vi "Get parameters from filename.vi"(0 "Filename":string="WS1021_PCB_01-03_VDD2p50CP17_R2-074200_R3-074302.s2p_right_DUT", 1 "File name format":T1, 3 "Comment lines":string[](array[string]), 5 "Idd":dbl, 9 "extension":string, 11 "Error In":errorcluster) -> (4 "Heading":string[](array[string]), 6 "Info":string[](array[string]), 10 "Registers":string[][](array[string]), 12 "Vdd (V)":dbl, 15 "Error Out":errorcluster)   [LabVIEW 2020]
uses:
  File Name Format.ctl
panel:
  out "CPV 2":i32(ring)=17 items=["CP 24V", "CP 26V", "CP 28V", "CP 30V", "CP 31V", "CP 32V", "CP 33V", "CP 34V", "CP 35V", "CP 36V", "CP 37V", "CP 38V", "CP 39V", "CP 40V", "CP 41V", "CP 42V", "CP 43V", "CP 44V", "CP 45V", "CP 46V", "CP 47V", "CP 48V", "CP 49V", "CP 50V", "CP 51V", "CP 52V", "CP 53V", "CP 54V", "CP 56V", "CP 58V", "CP 60V", "CP 62V"]
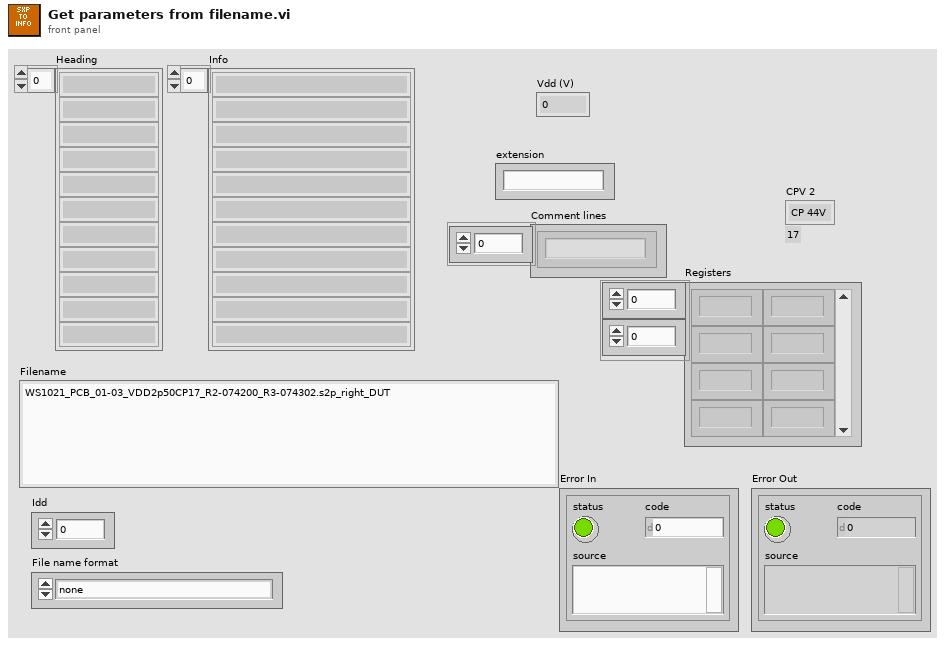
[diagram p1: front panel]
types:
  T1 = typedef "File Name Format.ctl" = enum16{"none", "S-para, old", "S-para, new", "S-para, new, step", "ECP", "S-para, new+1", "WS1040", "S-para, new+5100", "S-para, new+5100, no step", "General, space limited", "General, underscore limited", "General, whitespace limited", "LV-framework", "LV-framework, no file name"}
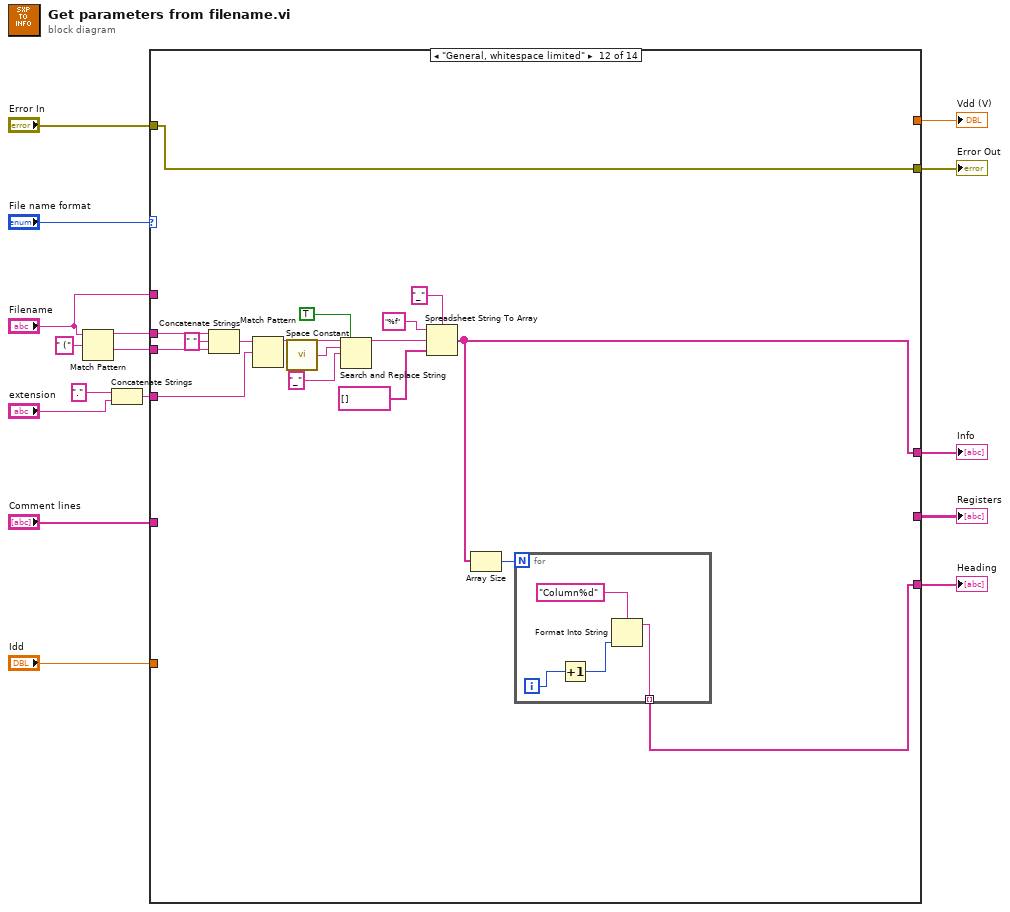
[diagram p0: block diagram]
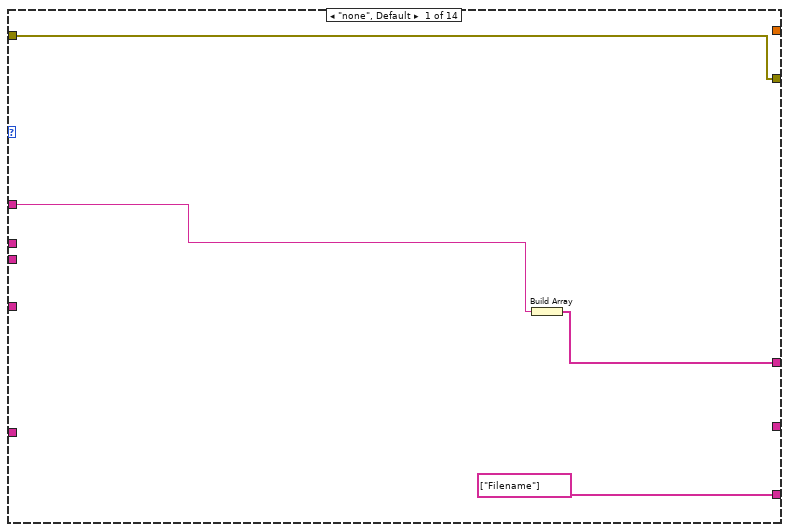
[diagram p2: hidden frame]
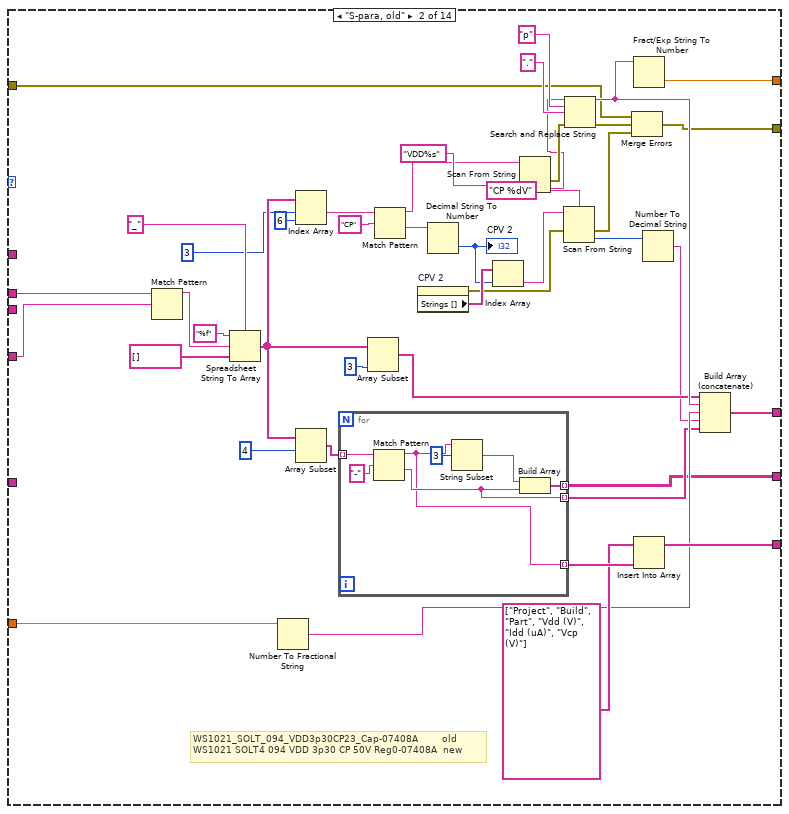
[diagram p3: hidden frame]
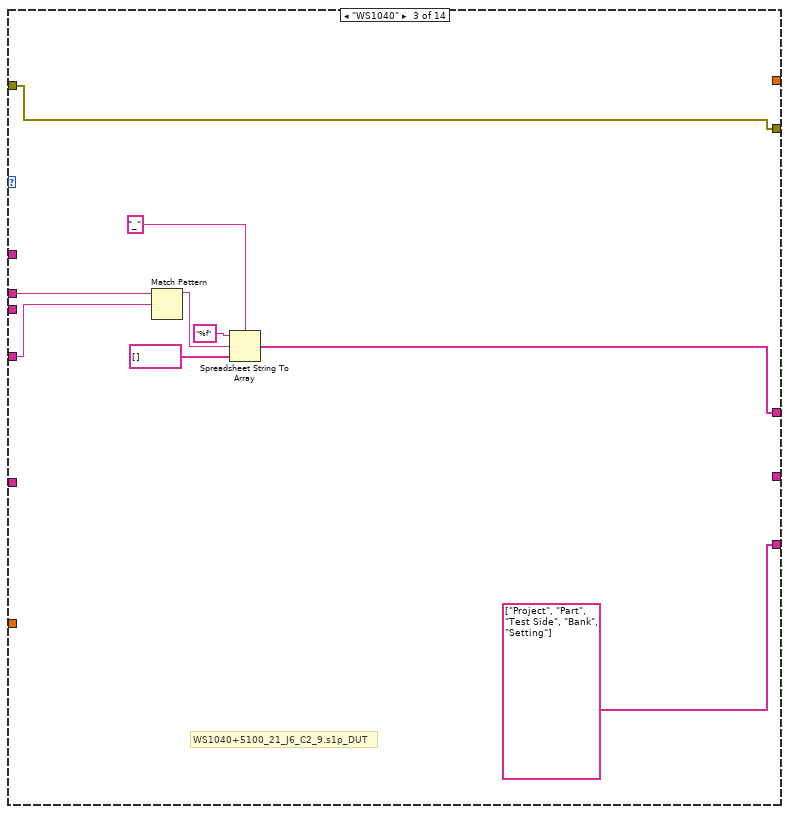
[diagram p4: hidden frame]
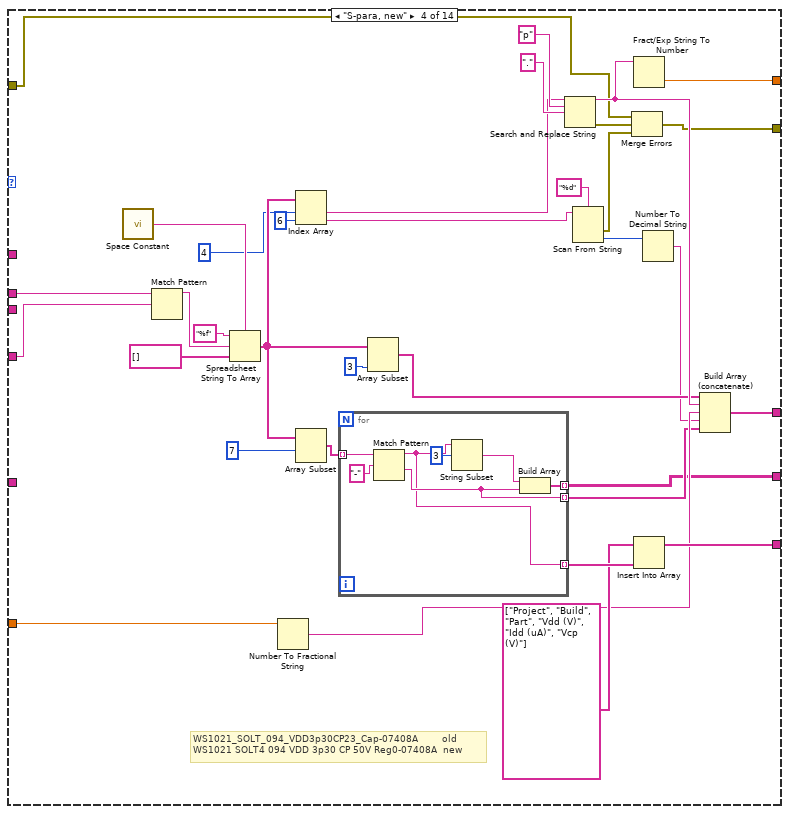
[diagram p5: hidden frame]
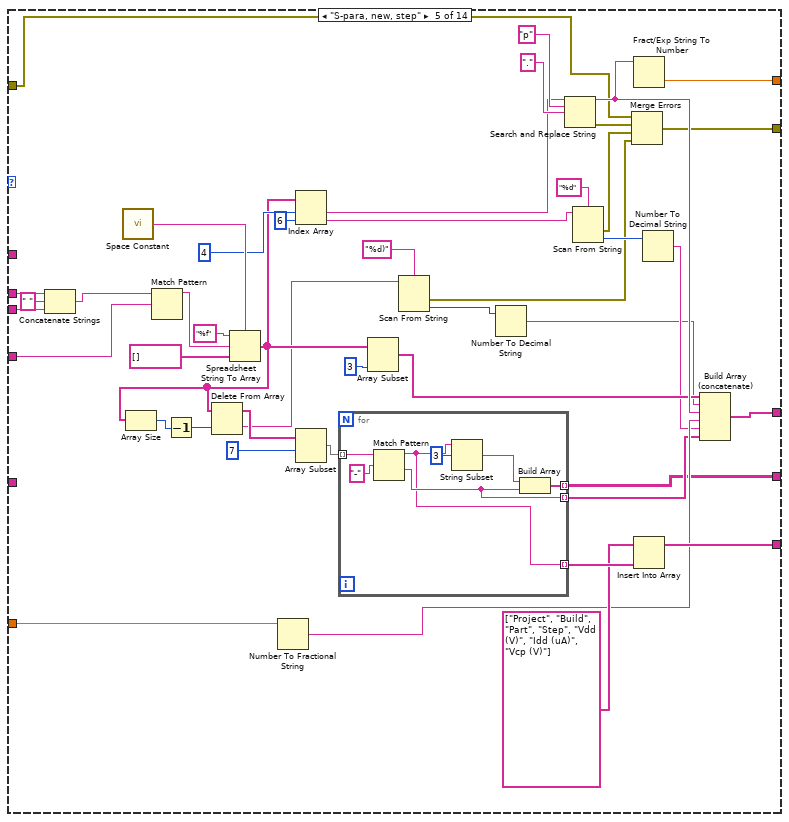
[diagram p6: hidden frame]
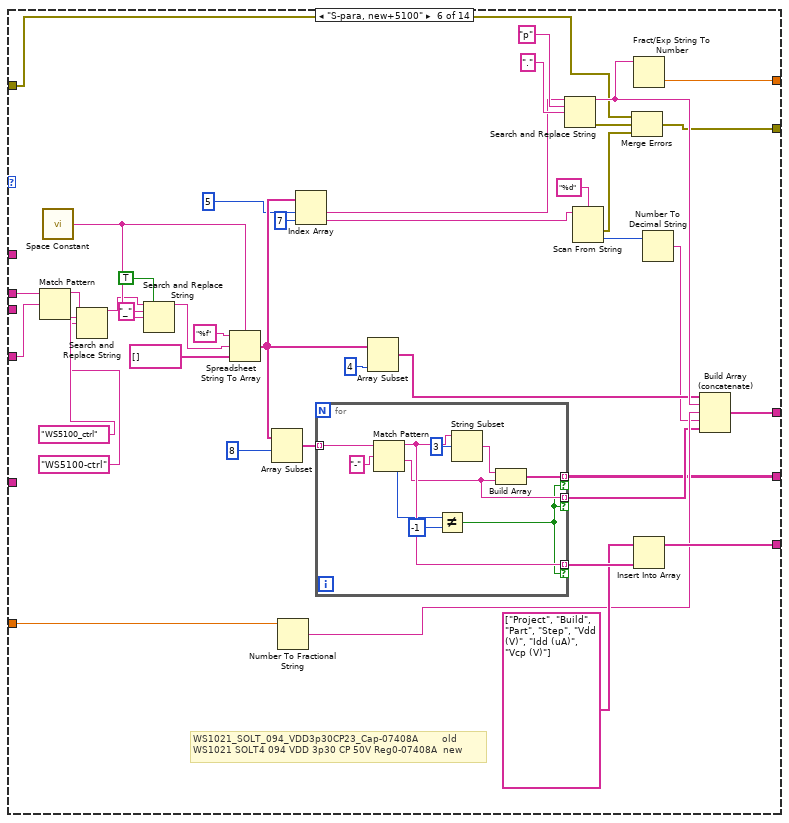
[diagram p7: hidden frame]
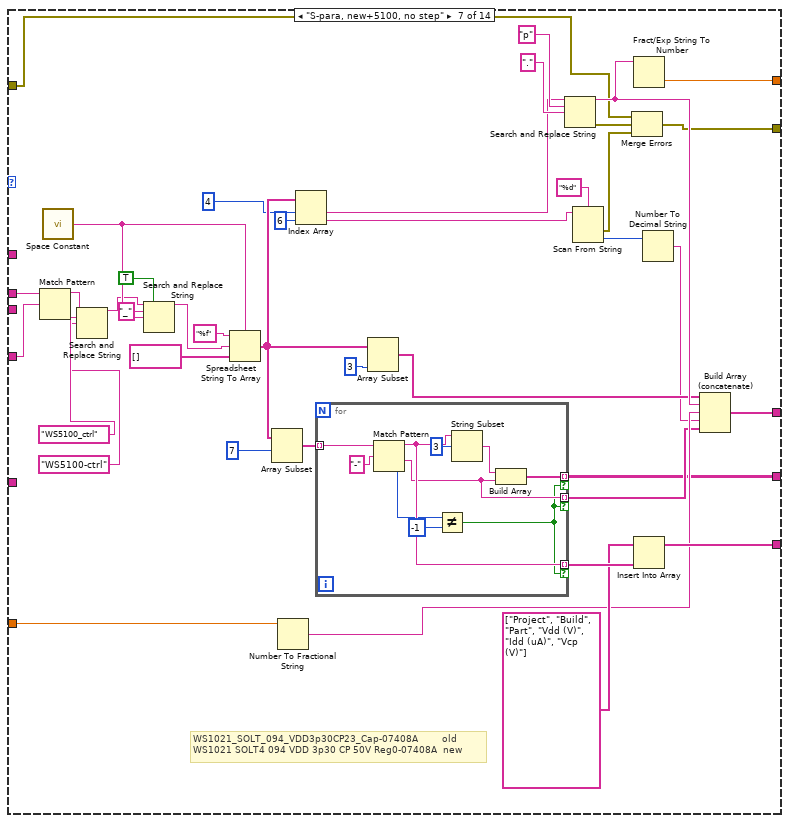
[diagram p8: hidden frame]
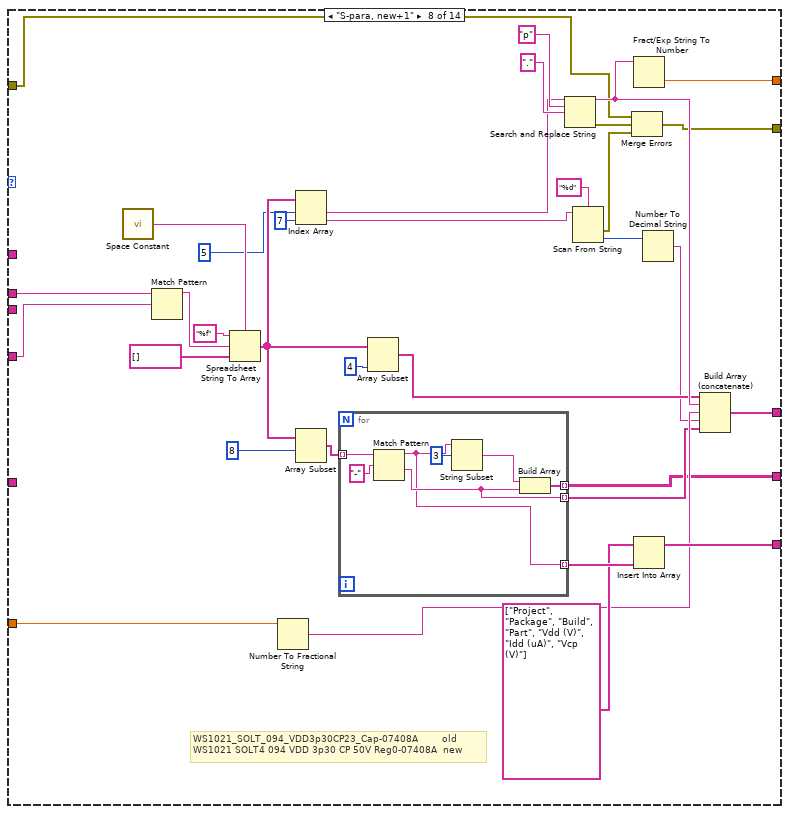
[diagram p9: hidden frame]
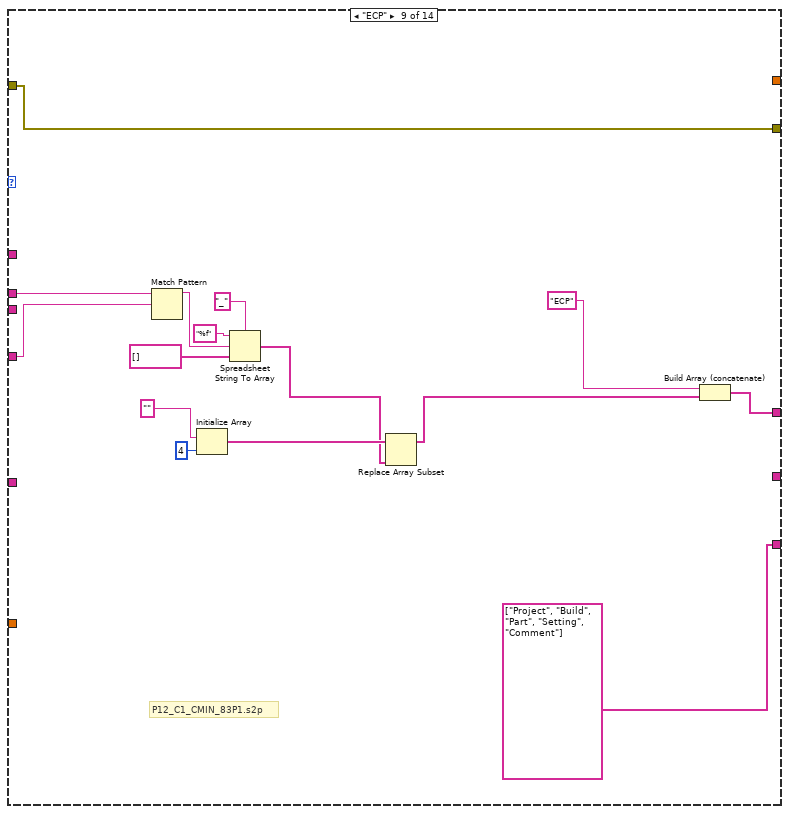
[diagram p10: hidden frame]
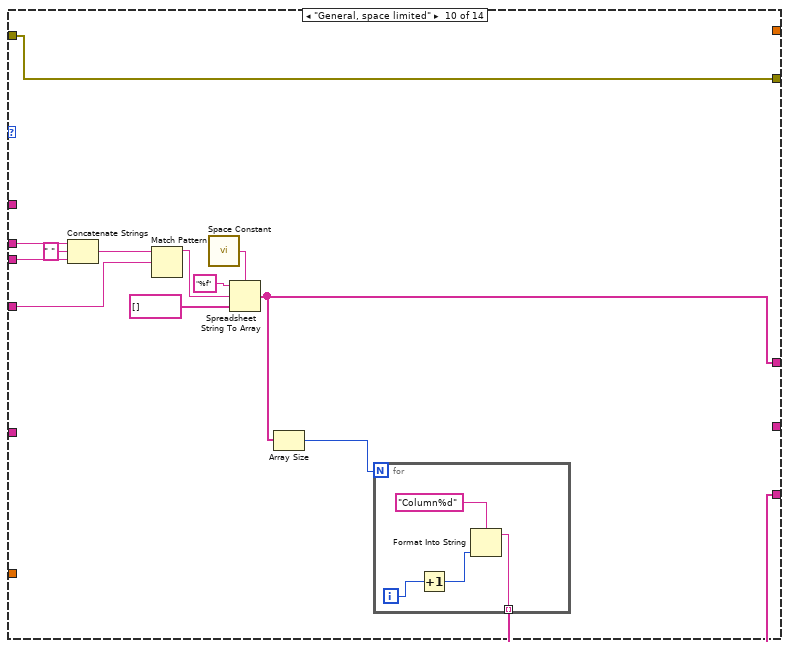
[diagram p11: hidden frame]
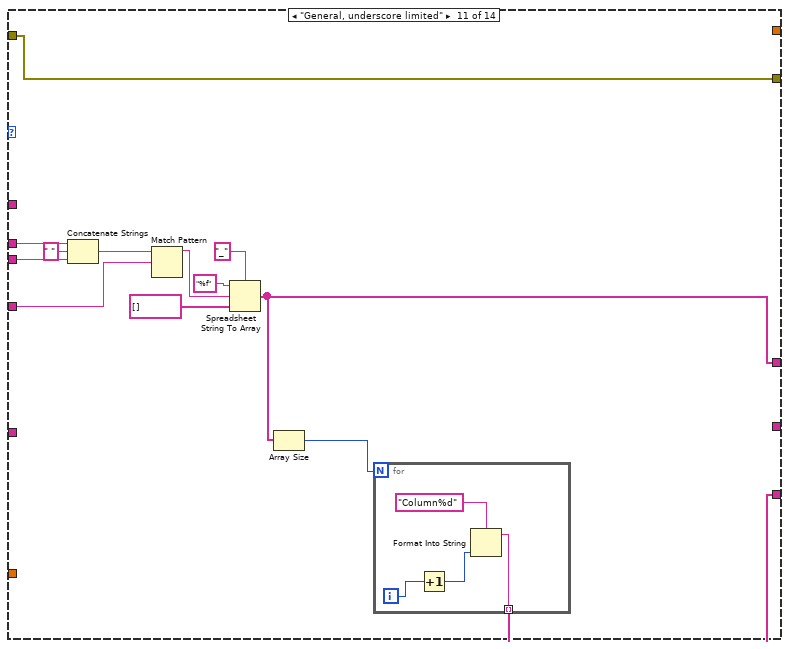
[diagram p12: hidden frame]
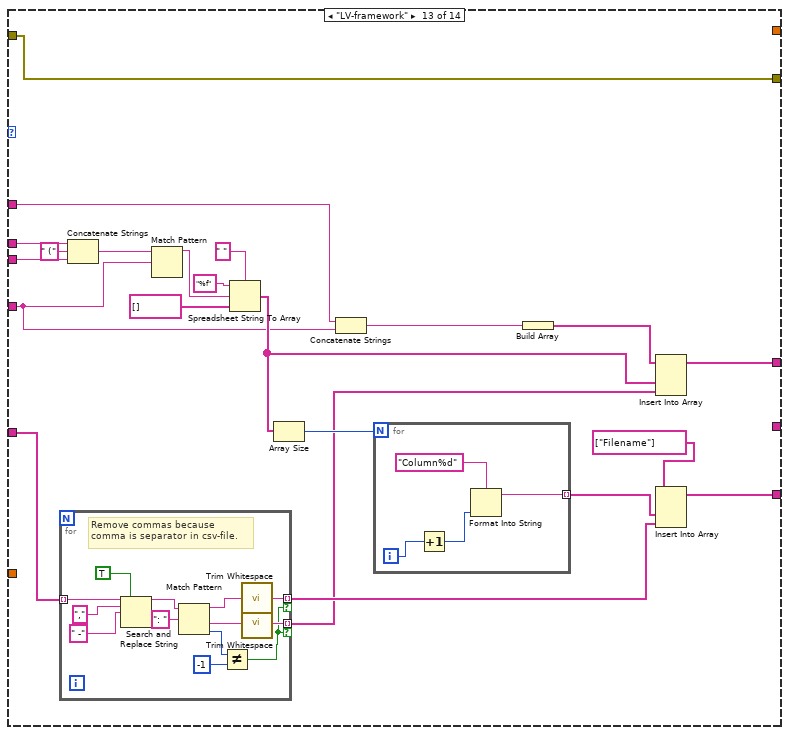
[diagram p13: hidden frame]
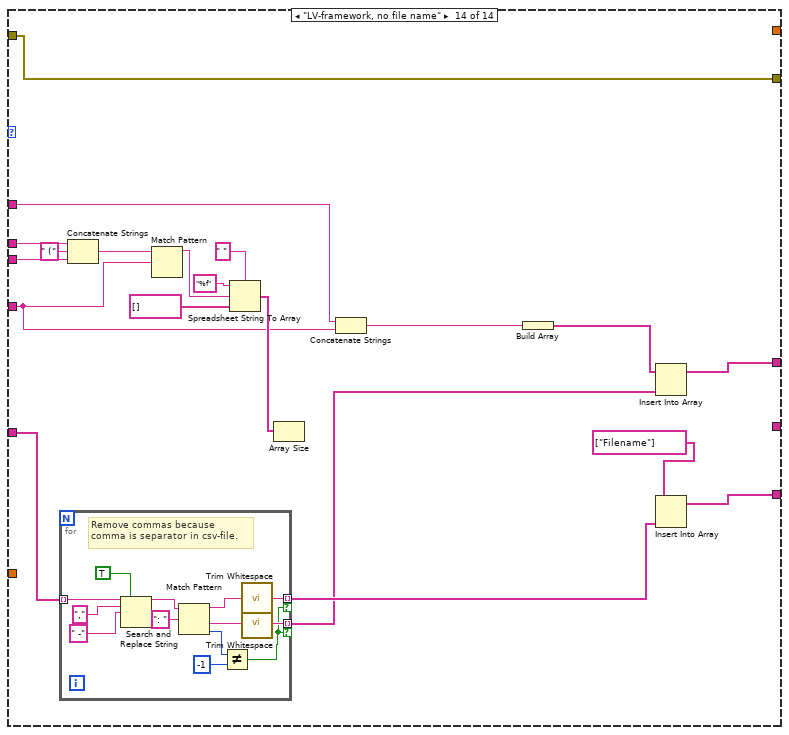
[diagram p14: hidden frame]
diagram:
  n1 = Match Pattern(string="Filename", regular expression=" (") -> (before substring=w7:string, after substring=w5:string)  [unwired: 1 in, 2 out]
  n2 = Concatenate Strings("." ("string"), "extension") -> (w9:string)
  n3 = case shown="\"General, whitespace limited\"" "File name format" {
    tunnel: [_ w59 _ w109 w161 w208 w258 w302 _ _ _ _ _ _] -> w16
    tunnel: [string[] ["Filename"] w51 string[] ["Project", "Part", "Test Side", "Bank", "Setting"] w102 w155 w202 w252 w295 string[] ["Project", "Build", "Part", "Setting", "Comment"] w329 w346 w368 w392 w431] -> w2
    tunnel: [w19 w48 w76 w99 w152 w199 w249 w292 w324 w331 w348 w370 w394 w433] -> w3
    tunnel: [w18 w46 w72 w97 w150 w197 w247 w290 w315 w337 w354 w376 w401 w438] -> w15
    tunnel: w7 -> [_ w34 w73 w85 w132 w186 w236 w278 w322 w334 w351 w373 w399 w426]
    tunnel: "Idd" -> [_ w24 _ w83 w137 w184 w234 w276 _ _ _ _ _ _]
    tunnel: "Error In" -> [w18 w23 w72 w82 w136 w183 w233 w275 w315 w337 w354 w376 w401 w438]
    tunnel: [_ w22 _ w81 w135 w182 w232 w274 _ _ _ _ _ _] -> w11
    tunnel: w9 -> [_ w21 w71 w80 w134 w181 w231 w273 w314 w336 w353 w375 w387 w427]
    tunnel: w5 -> [_ _ _ _ w133 _ _ _ _ w333 w350 w372 w398 w436]
    tunnel: "Comment lines" -> [_ _ _ _ _ _ _ _ _ _ _ _ w396 w435]
    tunnel: "Filename" -> [w17 _ _ _ _ _ _ _ _ _ _ _ w385 w424]
    frame "none", Default {
      n4 = Build Array(w17) -> (w19:string[])
    }
    frame "S-para, old" {
      # "WS1021_SOLT_094_VDD3p30CP23_Cap-07408A        old\nWS1021 SOLT4 094 VDD 3p30 CP 50V Reg0-07408A  new"
      n5 = Match Pattern(string=w34, regular expression=w21) -> (before substring=w58:string)  [unwired: 1 in, 3 out]
      n6 = Spreadsheet String To Array(delimiter (Tab)="_", format string="%f", spreadsheet string=w58, array type (2D Dbl)=string[] []) -> (array=w55:string[])
      n7 = Number To Fractional String(number=w24) -> (F-format string=w44:string)  [unwired: 3 in]
      n8 = Index Array(array=w55, index #1=3 ("index"), index #2=6 ("index")) -> (element #1=w57:string)  [unwired: 1 out]
      n9 = Array Subset(array=w55, index=4) -> (w56:string[])  [unwired: 1 in]
      n10 = for {
        tunnel: w56 -> [w69] mode=indexing
        tunnel: [w70] -> w22 mode=indexing
        tunnel: [w66] -> w53 mode=indexing
        tunnel: [w67] -> w43 mode=indexing
        n11 = Match Pattern(string=w69, regular expression="-") -> (before substring=w66:string, after substring=w67:string)  [unwired: 1 in, 2 out]
        n12 = String Subset(string=w66, offset (0)=3) -> (substring=w64:string)  [unwired: 1 in]
        n13 = Build Array(w64, w67) -> (w70:string[])
      }
      n14 = Array Subset(array=w55, length=3 ("index")) -> (w49:string[])  [unwired: 1 in]
      n15 = Match Pattern(string=w57, regular expression="CP") -> (before substring=w25:string, after substring=w32:string)  [unwired: 1 in, 2 out]
      n16 = property on="CPV 2" class="Ring (strict)"() -> (error out=w29:errorcluster, "Strings []"=w31:string[])  [unwired: 2 in, 1 out]
      n17 = Decimal String To Number(string=w32) -> (number=w30:i32)  [unwired: 2 in, 1 out]
      "CPV 2" <- w30
      n18 = Index Array(array=w31, index=w30) -> (element=w27:string)
      n19 = Scan From String(format string="VDD%s", input string=w25) -> (error out=w39:errorcluster, output 1=w38:string)  [unwired: 3 in, 2 out]
      n20 = Scan From String(format string="CP %dV", input string=w27, error in=w29) -> (error out=w45:errorcluster, output 1=w36:i32)  [unwired: 2 in, 2 out]
      n21 = Search and Replace String(input string=w38, search string="p", replace string="." ("replace string (\"\")"), error in=w39) -> (result string=w50:string, error out=w47:errorcluster)  [unwired: 4 in, 2 out]
      n22 = Merge Errors(w23, w47, w45) -> (w46:errorcluster)
      n23 = Fract/Exp String To Number(string=w50) -> (number=w59:dbl)  [unwired: 3 in, 1 out]
      n24 = Insert Into Array(array=string[] ["Project", "Build", "Part", "Vdd (V)", "Idd (uA)", "Vcp (V)"], new element=w53) -> (w51:string[])  [unwired: 1 in]
      n25 = Number To Decimal String(number=w36) -> (decimal integer string=w35:string)  [unwired: 1 in]
      n26 = Build Array (concatenate)(w49, w50, w44, w35, w43) -> (w48:string[])
    }
    frame "WS1040" {
      # "WS1040+5100_21_J6_C2_9.s1p_DUT"
      n27 = Match Pattern(string=w73, regular expression=w71) -> (before substring=w77:string)  [unwired: 1 in, 3 out]
      n28 = Spreadsheet String To Array(delimiter (Tab)="_", format string="%f", spreadsheet string=w77, array type (2D Dbl)=string[] []) -> (array=w76:string[])
    }
    frame "S-para, new" {
      # "WS1021_SOLT_094_VDD3p30CP23_Cap-07408A        old\nWS1021 SOLT4 094 VDD 3p30 CP 50V Reg0-07408A  new"
      n29 = call <vilib>:"Space Constant.vi"() -> ("String"=w93:string)
      n30 = Match Pattern(string=w85, regular expression=w80) -> (before substring=w108:string)  [unwired: 1 in, 3 out]
      n31 = Spreadsheet String To Array(delimiter (Tab)=w93, format string="%f", spreadsheet string=w108, array type (2D Dbl)=string[] []) -> (array=w106:string[])
      n32 = Number To Fractional String(number=w83) -> (F-format string=w95:string)  [unwired: 3 in]
      n33 = Index Array(array=w106, index #1=4 ("index"), index #2=6 ("index")) -> (element #1=w90:string, element #2=w88:string)
      n34 = Array Subset(array=w106, index=7) -> (w107:string[])  [unwired: 1 in]
      n35 = for {
        tunnel: w107 -> [w119] mode=indexing
        tunnel: [w120] -> w81 mode=indexing
        tunnel: [w116] -> w104 mode=indexing
        tunnel: [w117] -> w94 mode=indexing
        n36 = Match Pattern(string=w119, regular expression="-") -> (before substring=w116:string, after substring=w117:string)  [unwired: 1 in, 2 out]
        n37 = String Subset(string=w116, offset (0)=3) -> (substring=w114:string)  [unwired: 1 in]
        n38 = Build Array(w114, w117) -> (w120:string[])
      }
      n39 = Array Subset(array=w106, length=3 ("index")) -> (w100:string[])  [unwired: 1 in]
      n40 = Search and Replace String(input string=w90, search string="p", replace string="." ("replace string (\"\")")) -> (result string=w101:string, error out=w98:errorcluster)  [unwired: 5 in, 2 out]
      n41 = Scan From String(format string="%d", input string=w88) -> (error out=w96:errorcluster, output 1=w87:i32)  [unwired: 3 in, 2 out]
      n42 = Merge Errors(w82, w98, w96) -> (w97:errorcluster)
      n43 = Fract/Exp String To Number(string=w101) -> (number=w109:dbl)  [unwired: 3 in, 1 out]
      n44 = Insert Into Array(array=string[] ["Project", "Build", "Part", "Vdd (V)", "Idd (uA)", "Vcp (V)"], new element=w104) -> (w102:string[])  [unwired: 1 in]
      n45 = Number To Decimal String(number=w87) -> (decimal integer string=w86:string)  [unwired: 1 in]
      n46 = Build Array (concatenate)(w100, w101, w95, w86, w94) -> (w99:string[])
    }
    frame "S-para, new, step" {
      n47 = Concatenate Strings(w132, " " ("string"), w133) -> (w131:string)
      n48 = call <vilib>:"Space Constant.vi"() -> ("String"=w146:string)
      n49 = Match Pattern(string=w131, regular expression=w134) -> (before substring=w160:string)  [unwired: 1 in, 3 out]
      n50 = Spreadsheet String To Array(delimiter (Tab)=w146, format string="%f", spreadsheet string=w160, array type (2D Dbl)=string[] []) -> (array=w128:string[])
      n51 = Array Size(array=w128) -> (size(s)=w127:i32)
      n52 = Decrement(x=w127) -> (x-1=w126:i32)
      n53 = Delete From Array(array=w128, index=w126) -> (deleted portion=w125:string, array with subset deleted=w129:string[])  [unwired: 1 in]
      n54 = Number To Fractional String(number=w137) -> (F-format string=w148:string)  [unwired: 3 in]
      n55 = Index Array(array=w128, index #1=4 ("index"), index #2=6 ("index")) -> (element #1=w143:string, element #2=w141:string)
      n56 = Array Subset(array=w129, index=7) -> (w159:string[])  [unwired: 1 in]
      n57 = for {
        tunnel: w159 -> [w171] mode=indexing
        tunnel: [w172] -> w135 mode=indexing
        tunnel: [w168] -> w157 mode=indexing
        tunnel: [w169] -> w147 mode=indexing
        n58 = Match Pattern(string=w171, regular expression="-") -> (before substring=w168:string, after substring=w169:string)  [unwired: 1 in, 2 out]
        n59 = String Subset(string=w168, offset (0)=3) -> (substring=w166:string)  [unwired: 1 in]
        n60 = Build Array(w166, w169) -> (w172:string[])
      }
      n61 = Array Subset(array=w128, length=3 ("index")) -> (w153:string[])  [unwired: 1 in]
      n62 = Scan From String(format string="%d)", input string=w125) -> (error out=w121:errorcluster, output 1=w123:i32)  [unwired: 3 in, 2 out]
      n63 = Number To Decimal String(number=w123) -> (decimal integer string=w122:string)  [unwired: 1 in]
      n64 = Search and Replace String(input string=w143, search string="p", replace string="." ("replace string (\"\")")) -> (result string=w154:string, error out=w151:errorcluster)  [unwired: 5 in, 2 out]
      n65 = Scan From String(format string="%d", input string=w141) -> (error out=w149:errorcluster, output 1=w140:i32)  [unwired: 3 in, 2 out]
      n66 = Merge Errors(w136, w151, w149, w121) -> (w150:errorcluster)
      n67 = Fract/Exp String To Number(string=w154) -> (number=w161:dbl)  [unwired: 3 in, 1 out]
      n68 = Insert Into Array(array=string[] ["Project", "Build", "Part", "Step", "Vdd (V)", "Idd (uA)", "Vcp (V)"], new element=w157) -> (w155:string[])  [unwired: 1 in]
      n69 = Number To Decimal String(number=w140) -> (decimal integer string=w139:string)  [unwired: 1 in]
      n70 = Build Array (concatenate)(w153, w122, w154, w148, w139, w147) -> (w152:string[])
    }
    frame "S-para, new+5100" {
      # "WS1021_SOLT_094_VDD3p30CP23_Cap-07408A        old\nWS1021 SOLT4 094 VDD 3p30 CP 50V Reg0-07408A  new"
      n71 = Match Pattern(string=w186, regular expression=w181) -> (before substring=w176:string)  [unwired: 1 in, 3 out]
      n72 = call <vilib>:"Space Constant.vi"() -> ("String"=w179:string)
      n73 = Search and Replace String(input string=w176, search string="WS5100_ctrl" ("format string"), replace string="WS5100-ctrl" ("format string")) -> (result string=w175:string)  [unwired: 5 in, 3 out]
      n74 = Search and Replace String(replace all?=TRUE ("replace all? (F)"), input string=w175, search string="_", replace string=w179) -> (result string=w180:string)  [unwired: 4 in, 3 out]
      n75 = Spreadsheet String To Array(delimiter (Tab)=w179, format string="%f", spreadsheet string=w180, array type (2D Dbl)=string[] []) -> (array=w206:string[])
      n76 = Array Subset(array=w206, index=8) -> (w207:string[])  [unwired: 1 in]
      n77 = Number To Fractional String(number=w184) -> (F-format string=w195:string)  [unwired: 3 in]
      n78 = Index Array(array=w206, index #1=5 ("index"), index #2=7 ("index")) -> (element #1=w191:string, element #2=w189:string)
      n79 = for {
        tunnel: w207 -> [w221] mode=indexing
        tunnel: [w222] -> w182 mode=indexing if=w213
        tunnel: [w219] -> w204 mode=indexing if=w213
        tunnel: [w216] -> w194 mode=indexing if=w213
        n80 = Match Pattern(string=w221, regular expression="-") -> (before substring=w219:string, after substring=w216:string, offset past match=w215:i32)  [unwired: 1 in, 1 out]
        n81 = Not Equal?(x=w215, y=-1) -> (x != y?=w213:bool)
        n82 = String Subset(string=w219, offset (0)=3) -> (substring=w217:string)  [unwired: 1 in]
        n83 = Build Array(w217, w216) -> (w222:string[])
      }
      n84 = Array Subset(array=w206, length=4 ("index")) -> (w200:string[])  [unwired: 1 in]
      n85 = Search and Replace String(input string=w191, search string="p", replace string="." ("replace string (\"\")")) -> (result string=w201:string, error out=w198:errorcluster)  [unwired: 5 in, 2 out]
      n86 = Scan From String(format string="%d", input string=w189) -> (error out=w196:errorcluster, output 1=w188:i32)  [unwired: 3 in, 2 out]
      n87 = Merge Errors(w183, w198, w196) -> (w197:errorcluster)
      n88 = Fract/Exp String To Number(string=w201) -> (number=w208:dbl)  [unwired: 3 in, 1 out]
      n89 = Insert Into Array(array=string[] ["Project", "Build", "Part", "Step", "Vdd (V)", "Idd (uA)", "Vcp (V)"], new element=w204) -> (w202:string[])  [unwired: 1 in]
      n90 = Number To Decimal String(number=w188) -> (decimal integer string=w187:string)  [unwired: 1 in]
      n91 = Build Array (concatenate)(w200, w201, w195, w187, w194) -> (w199:string[])
    }
    frame "S-para, new+5100, no step" {
      # "WS1021_SOLT_094_VDD3p30CP23_Cap-07408A        old\nWS1021 SOLT4 094 VDD 3p30 CP 50V Reg0-07408A  new"
      n92 = Match Pattern(string=w236, regular expression=w231) -> (before substring=w226:string)  [unwired: 1 in, 3 out]
      n93 = call <vilib>:"Space Constant.vi"() -> ("String"=w229:string)
      n94 = Search and Replace String(input string=w226, search string="WS5100_ctrl" ("format string"), replace string="WS5100-ctrl" ("format string")) -> (result string=w225:string)  [unwired: 5 in, 3 out]
      n95 = Search and Replace String(replace all?=TRUE ("replace all? (F)"), input string=w225, search string="_", replace string=w229) -> (result string=w230:string)  [unwired: 4 in, 3 out]
      n96 = Spreadsheet String To Array(delimiter (Tab)=w229, format string="%f", spreadsheet string=w230, array type (2D Dbl)=string[] []) -> (array=w256:string[])
      n97 = Array Subset(array=w256, index=7) -> (w257:string[])  [unwired: 1 in]
      n98 = Number To Fractional String(number=w234) -> (F-format string=w245:string)  [unwired: 3 in]
      n99 = Index Array(array=w256, index #1=4 ("index"), index #2=6 ("index")) -> (element #1=w241:string, element #2=w239:string)
      n100 = for {
        tunnel: w257 -> [w271] mode=indexing
        tunnel: [w272] -> w232 mode=indexing if=w263
        tunnel: [w269] -> w254 mode=indexing if=w263
        tunnel: [w266] -> w244 mode=indexing if=w263
        n101 = Match Pattern(string=w271, regular expression="-") -> (before substring=w269:string, after substring=w266:string, offset past match=w265:i32)  [unwired: 1 in, 1 out]
        n102 = Not Equal?(x=w265, y=-1) -> (x != y?=w263:bool)
        n103 = String Subset(string=w269, offset (0)=3) -> (substring=w267:string)  [unwired: 1 in]
        n104 = Build Array(w267, w266) -> (w272:string[])
      }
      n105 = Array Subset(array=w256, length=3 ("index")) -> (w250:string[])  [unwired: 1 in]
      n106 = Search and Replace String(input string=w241, search string="p", replace string="." ("replace string (\"\")")) -> (result string=w251:string, error out=w248:errorcluster)  [unwired: 5 in, 2 out]
      n107 = Scan From String(format string="%d", input string=w239) -> (error out=w246:errorcluster, output 1=w238:i32)  [unwired: 3 in, 2 out]
      n108 = Merge Errors(w233, w248, w246) -> (w247:errorcluster)
      n109 = Fract/Exp String To Number(string=w251) -> (number=w258:dbl)  [unwired: 3 in, 1 out]
      n110 = Insert Into Array(array=string[] ["Project", "Build", "Part", "Vdd (V)", "Idd (uA)", "Vcp (V)"], new element=w254) -> (w252:string[])  [unwired: 1 in]
      n111 = Number To Decimal String(number=w238) -> (decimal integer string=w237:string)  [unwired: 1 in]
      n112 = Build Array (concatenate)(w250, w251, w245, w237, w244) -> (w249:string[])
    }
    frame "S-para, new+1" {
      # "WS1021_SOLT_094_VDD3p30CP23_Cap-07408A        old\nWS1021 SOLT4 094 VDD 3p30 CP 50V Reg0-07408A  new"
      n113 = call <vilib>:"Space Constant.vi"() -> ("String"=w286:string)
      n114 = Match Pattern(string=w278, regular expression=w273) -> (before substring=w301:string)  [unwired: 1 in, 3 out]
      n115 = Spreadsheet String To Array(delimiter (Tab)=w286, format string="%f", spreadsheet string=w301, array type (2D Dbl)=string[] []) -> (array=w299:string[])
      n116 = Number To Fractional String(number=w276) -> (F-format string=w288:string)  [unwired: 3 in]
      n117 = Index Array(array=w299, index #1=5 ("index"), index #2=7 ("index")) -> (element #1=w283:string, element #2=w281:string)
      n118 = Array Subset(array=w299, index=8) -> (w300:string[])  [unwired: 1 in]
      n119 = for {
        tunnel: w300 -> [w312] mode=indexing
        tunnel: [w313] -> w274 mode=indexing
        tunnel: [w309] -> w297 mode=indexing
        tunnel: [w310] -> w287 mode=indexing
        n120 = Match Pattern(string=w312, regular expression="-") -> (before substring=w309:string, after substring=w310:string)  [unwired: 1 in, 2 out]
        n121 = String Subset(string=w309, offset (0)=3) -> (substring=w307:string)  [unwired: 1 in]
        n122 = Build Array(w307, w310) -> (w313:string[])
      }
      n123 = Array Subset(array=w299, length=4 ("index")) -> (w293:string[])  [unwired: 1 in]
      n124 = Search and Replace String(input string=w283, search string="p", replace string="." ("replace string (\"\")")) -> (result string=w294:string, error out=w291:errorcluster)  [unwired: 5 in, 2 out]
      n125 = Scan From String(format string="%d", input string=w281) -> (error out=w289:errorcluster, output 1=w280:i32)  [unwired: 3 in, 2 out]
      n126 = Merge Errors(w275, w291, w289) -> (w290:errorcluster)
      n127 = Fract/Exp String To Number(string=w294) -> (number=w302:dbl)  [unwired: 3 in, 1 out]
      n128 = Insert Into Array(array=string[] ["Project", "Package", "Build", "Part", "Vdd (V)", "Idd (uA)", "Vcp (V)"], new element=w297) -> (w295:string[])  [unwired: 1 in]
      n129 = Number To Decimal String(number=w280) -> (decimal integer string=w279:string)  [unwired: 1 in]
      n130 = Build Array (concatenate)(w293, w294, w288, w279, w287) -> (w292:string[])
    }
    frame "ECP" {
      # "P12_C1_CMIN_83P1.s2p"
      n131 = Match Pattern(string=w322, regular expression=w314) -> (before substring=w326:string)  [unwired: 1 in, 3 out]
      n132 = Initialize Array("" ("delimiter (Tab)"), 4 ("dimension size")) -> (w318:string[])
      n133 = Spreadsheet String To Array(delimiter (Tab)="_", format string="%f", spreadsheet string=w326, array type (2D Dbl)=string[] []) -> (array=w317:string[])
      n134 = Replace Array Subset(array=w318, new element=w317) -> (w316:string[])  [unwired: 1 in]
      n135 = Build Array (concatenate)("ECP" ("result string"), w316) -> (w324:string[])
    }
    frame "General, space limited" {
      n136 = Concatenate Strings(w334, " " ("string"), w333) -> (w332:string)
      n137 = Match Pattern(string=w332, regular expression=w336) -> (before substring=w339:string)  [unwired: 1 in, 3 out]
      n138 = call <vilib>:"Space Constant.vi"() -> ("String"=w338:string)
      n139 = Spreadsheet String To Array(delimiter (Tab)=w338, format string="%f", spreadsheet string=w339, array type (2D Dbl)=string[] []) -> (array=w331:string[])
      n140 = Array Size(array=w331) -> (size(s)=w330:i32)
      n141 = for {
        N: w330 -> [_]
        tunnel: [w342] -> w329 mode=indexing
        i -> [w344]
        n142 = Increment(x=w344) -> (x+1=w343:i32)
        n143 = Format Into String(format string="Column%d", w343) -> (resulting string=w342:string)  [unwired: 2 in, 1 out]
      }
    }
    frame "General, underscore limited" {
      n144 = Concatenate Strings(w351, " " ("string"), w350) -> (w349:string)
      n145 = Match Pattern(string=w349, regular expression=w353) -> (before substring=w356:string)  [unwired: 1 in, 3 out]
      n146 = Spreadsheet String To Array(delimiter (Tab)="_", format string="%f", spreadsheet string=w356, array type (2D Dbl)=string[] []) -> (array=w348:string[])
      n147 = Array Size(array=w348) -> (size(s)=w347:i32)
      n148 = for {
        N: w347 -> [_]
        tunnel: [w359] -> w346 mode=indexing
        i -> [w361]
        n149 = Increment(x=w361) -> (x+1=w360:i32)
        n150 = Format Into String(format string="Column%d", w360) -> (resulting string=w359:string)  [unwired: 2 in, 1 out]
      }
    }
    frame "General, whitespace limited" {
      n151 = Concatenate Strings(w373, " " ("string"), w372) -> (w371:string)
      n152 = Match Pattern(string=w371, regular expression=w375) -> (before substring=w367:string)  [unwired: 1 in, 3 out]
      n153 = call <vilib>:"Space Constant.vi"() -> ("String"=w364:string)
      n154 = Search and Replace String(replace all?=TRUE ("replace all? (F)"), input string=w367, search string=w364, replace string="_") -> (result string=w366:string)  [unwired: 4 in, 3 out]
      n155 = Spreadsheet String To Array(delimiter (Tab)="_", format string="%f", spreadsheet string=w366, array type (2D Dbl)=string[] []) -> (array=w370:string[])
      n156 = Array Size(array=w370) -> (size(s)=w369:i32)
      n157 = for {
        N: w369 -> [_]
        tunnel: [w380] -> w368 mode=indexing
        i -> [w382]
        n158 = Increment(x=w382) -> (x+1=w381:i32)
        n159 = Format Into String(format string="Column%d", w381) -> (resulting string=w380:string)  [unwired: 2 in, 1 out]
      }
    }
    frame "LV-framework" {
      n160 = for {
        tunnel: w396 -> [w410] mode=indexing
        tunnel: [w414] -> w395 mode=indexing if=w411
        tunnel: [w415] -> w393 mode=indexing if=w411
        # "Remove commas because \ncomma is separator in csv-file."
        n161 = Search and Replace String(replace all?=TRUE ("replace all? (F)"), input string=w410, search string=",", replace string=" -" ("replace string (\"\")")) -> (result string=w409:string)  [unwired: 4 in, 3 out]
        n162 = Match Pattern(string=w409, regular expression=": ") -> (before substring=w416:string, after substring=w417:string, offset past match=w413:i32)  [unwired: 1 in, 1 out]
        n163 = Not Equal?(x=w413, y=-1) -> (x != y?=w411:bool)
        n164 = call <vilib>:"Trim Whitespace.vi"("string"=w416) -> ("trimmed string"=w414:string)  [unwired: 1 in]
        n165 = call <vilib>:"Trim Whitespace.vi"("string"=w417) -> ("trimmed string"=w415:string)  [unwired: 1 in]
      }
      n166 = Concatenate Strings(w399, " (" ("string"), w398) -> (w384:string)
      n167 = Match Pattern(string=w384, regular expression=w387) -> (before substring=w403:string)  [unwired: 1 in, 3 out]
      n168 = Spreadsheet String To Array(delimiter (Tab)=" ", format string="%f", spreadsheet string=w403, array type (2D Dbl)=string[] []) -> (array=w390:string[])
      n169 = Array Size(array=w390) -> (size(s)=w397:i32)
      n170 = Concatenate Strings(w385, w387) -> (w386:string)
      n171 = for {
        N: w397 -> [_]
        tunnel: [w419] -> w391 mode=indexing
        i -> [w421]
        n172 = Increment(x=w421) -> (x+1=w420:i32)
        n173 = Format Into String(format string="Column%d", w420) -> (resulting string=w419:string)  [unwired: 2 in, 1 out]
      }
      n174 = Build Array(w386) -> (w388:string[])
      n175 = Insert Into Array(array=w388, new element #1=w390, new element #2=w393) -> (w394:string[])  [unwired: 1 in]
      n176 = Insert Into Array(array=string[] ["Filename"], new element #1=w391, new element #2=w395) -> (w392:string[])  [unwired: 1 in]
    }
    frame "LV-framework, no file name" {
      n177 = for {
        tunnel: w435 -> [w447] mode=indexing
        tunnel: [w451] -> w434 mode=indexing if=w448
        tunnel: [w452] -> w432 mode=indexing if=w448
        # "Remove commas because \ncomma is separator in csv-file."
        n178 = Search and Replace String(replace all?=TRUE ("replace all? (F)"), input string=w447, search string=",", replace string=" -" ("replace string (\"\")")) -> (result string=w446:string)  [unwired: 4 in, 3 out]
        n179 = Match Pattern(string=w446, regular expression=": ") -> (before substring=w453:string, after substring=w454:string, offset past match=w450:i32)  [unwired: 1 in, 1 out]
        n180 = Not Equal?(x=w450, y=-1) -> (x != y?=w448:bool)
        n181 = call <vilib>:"Trim Whitespace.vi"("string"=w453) -> ("trimmed string"=w451:string)  [unwired: 1 in]
        n182 = call <vilib>:"Trim Whitespace.vi"("string"=w454) -> ("trimmed string"=w452:string)  [unwired: 1 in]
      }
      n183 = Concatenate Strings(w426, " (" ("string"), w436) -> (w425:string)
      n184 = Match Pattern(string=w425, regular expression=w427) -> (before substring=w440:string)  [unwired: 1 in, 3 out]
      n185 = Spreadsheet String To Array(delimiter (Tab)=" ", format string="%f", spreadsheet string=w440, array type (2D Dbl)=string[] []) -> (array=w430:string[])
      n186 = Array Size(array=w430) -> ()  [unwired: 1 out]
      n187 = Concatenate Strings(w424, w427) -> (w423:string)
      n188 = Build Array(w423) -> (w428:string[])
      n189 = Insert Into Array(array=w428, new element=w432) -> (w433:string[])  [unwired: 1 in]
      n190 = Insert Into Array(array=string[] ["Filename"], new element=w434) -> (w431:string[])  [unwired: 1 in]
    }
  }
  "Info" <- w3
  "Vdd (V)" <- w16
  "Heading" <- w2
  "Error Out" <- w15
  "Registers" <- w11
